vi "Debug Server Launcher.vi"() -> ()   [LabVIEW 2017]
doc: "Splash screen for the Debug Server application"
panel:
  out "dot3 4":picture
  out "dot2 4":picture
  out "dot1 4":picture
  out "dot3 3":picture
  out "dot2 3":picture
  out "dot1 3":picture
  out "dot3 2":picture
  out "dot2 2":picture
  out "dot1 2":picture
  out "dot1":picture
  out "dot2":picture
  out "dot3":picture
  in  "error in (no error)":errorcluster
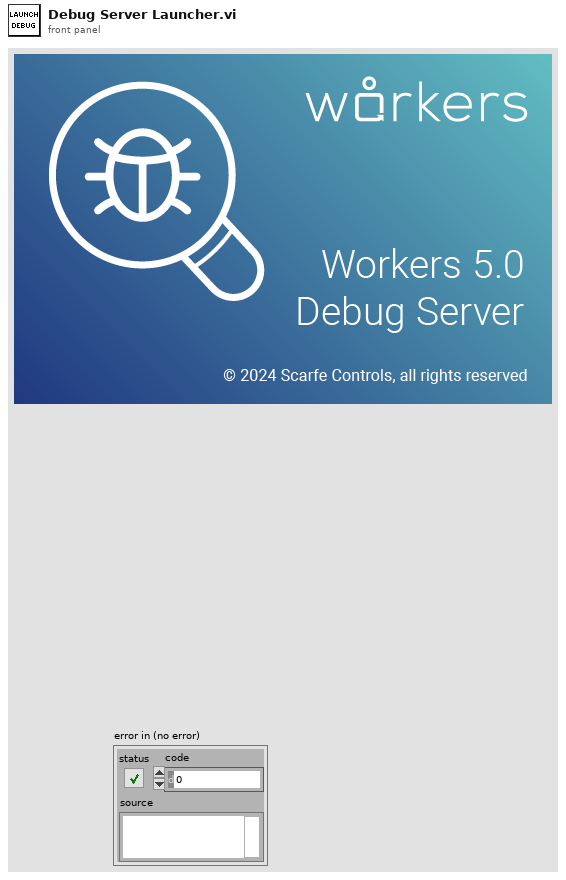
[diagram p1: front panel]
types:
  T1 = enum32{"Invalid", "Standard", "Closed", "Hidden", "Minimized", "Maximized"}
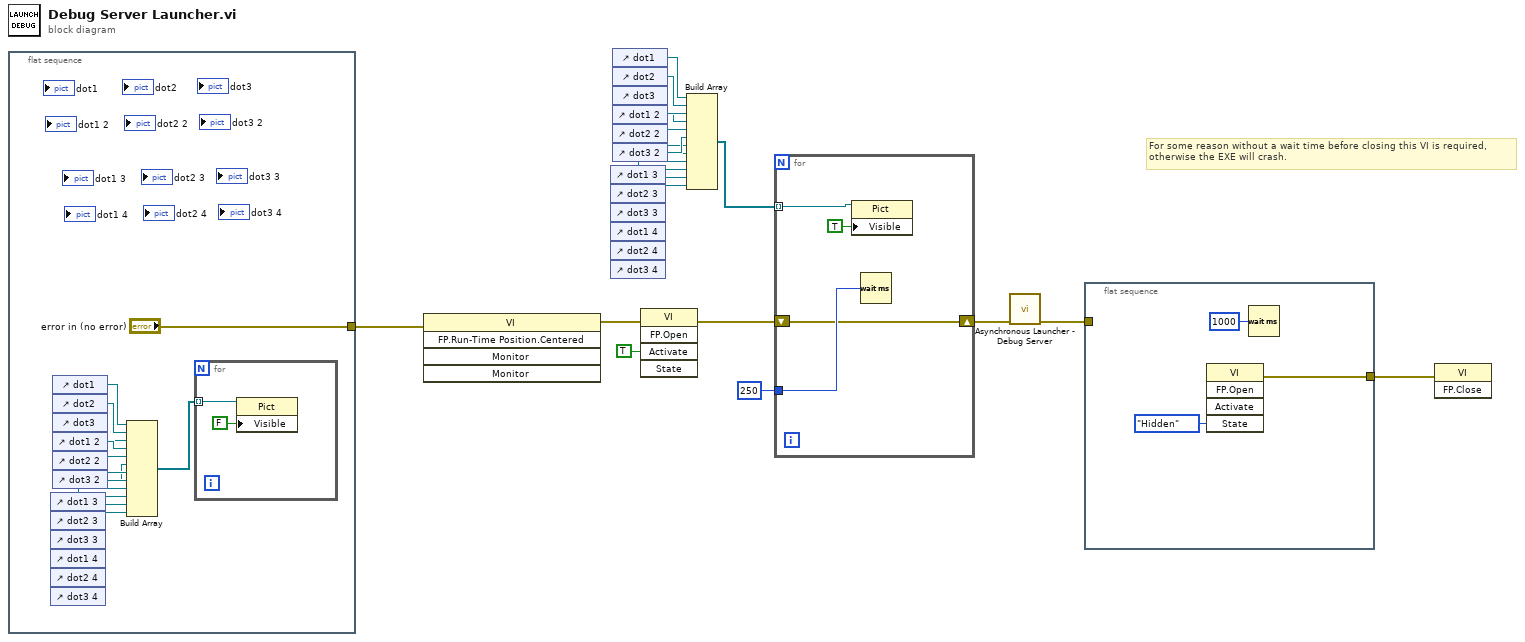
[diagram p0: block diagram]
diagram:
  # "For some reason without a wait time before closing this VI is required,\notherwise the EXE will crash."
  n1 = flat-sequence {
    tunnel: ["error in (no error)"] -> w21
    frame #0 {
      n2 = control-ref of="dot1 3"() -> (w29:refnum<vi>)
      n3 = control-ref of="dot2 3"() -> (w30:refnum<vi>)
      n4 = control-ref of="dot3 3"() -> (w31:refnum<vi>)
      n5 = control-ref of="dot1 4"() -> (w32:refnum<vi>)
      n6 = control-ref of="dot2 4"() -> (w33:refnum<vi>)
      n7 = control-ref of="dot3 4"() -> (w34:refnum<vi>)
      n8 = control-ref of="dot1"() -> (w23:refnum<vi>)
      n9 = control-ref of="dot2"() -> (w24:refnum<vi>)
      n10 = control-ref of="dot3"() -> (w25:refnum<vi>)
      n11 = control-ref of="dot1 2"() -> (w26:refnum<vi>)
      n12 = control-ref of="dot2 2"() -> (w27:refnum<vi>)
      n13 = control-ref of="dot3 2"() -> (w28:refnum<vi>)
      n14 = Build Array(w23, w24, w25, w26, w27, w28, w29, w30, w31, w32, w33, w34) -> (w22:refnum<vi>[])
      n15 = for {
        tunnel: w22 -> [w36] mode=indexing
        n16 = property class="Pict"(reference=w36, "Visible"=FALSE) -> ()  [unwired: 1 in, 2 out]
      }
    }
  }
  n17 = invoke class="VI" method="FP.Run-Time Position.Centered"(error in=w21) -> (error out=w20:errorcluster)  [unwired: 4 in, 4 out]
  n18 = control-ref of="dot1 3"() -> (w8:refnum<vi>)
  n19 = control-ref of="dot2 3"() -> (w7:refnum<vi>)
  n20 = control-ref of="dot3 3"() -> (w6:refnum<vi>)
  n21 = control-ref of="dot1 4"() -> (w5:refnum<vi>)
  n22 = control-ref of="dot2 4"() -> (w4:refnum<vi>)
  n23 = control-ref of="dot3 4"() -> (w3:refnum<vi>)
  n24 = control-ref of="dot1"() -> (w16:refnum<vi>)
  n25 = control-ref of="dot2"() -> (w15:refnum<vi>)
  n26 = control-ref of="dot3"() -> (w14:refnum<vi>)
  n27 = control-ref of="dot1 2"() -> (w13:refnum<vi>)
  n28 = control-ref of="dot2 2"() -> (w12:refnum<vi>)
  n29 = control-ref of="dot3 2"() -> (w11:refnum<vi>)
  n30 = invoke class="VI" method="FP.Open"(error in=w20, "Activate"=TRUE ("Activate?")) -> (error out=w9:errorcluster)  [unwired: 3 in, 4 out]
  n31 = Build Array(w16, w15, w14, w13, w12, w11, w8, w7, w6, w5, w4, w3) -> (w10:refnum<vi>[])
  n32 = for {
    tunnel: u32 250 ("milliseconds to wait") -> [w41]
    tunnel: w10 -> [w39] mode=indexing
    shift-right: [w38] -> w2
    shift-left: w9 -> [w38]
    n33 = property class="Pict"(reference=w39, "Visible"=TRUE) -> ()  [unwired: 1 in, 2 out]
    n34 = Wait (ms)(milliseconds to wait=w41) -> ()  [unwired: 1 out]
  }
  n35 = call "Asynchronous Launcher - Debug Server.vi"("error in"=w2) -> ("error out"=w1:errorcluster)  [unwired: 9 in, 1 out]
  n36 = flat-sequence {
    tunnel: [w43] -> w17
    tunnel: w1 -> [_]
    frame #0 {
      n37 = invoke class="VI" method="FP.Open"("State"=T1."Hidden") -> (error out=w43:errorcluster)  [unwired: 4 in, 4 out]
      n38 = Wait (ms)(milliseconds to wait=u32 1000) -> ()  [unwired: 1 out]
    }
  }
  n39 = invoke class="VI" method="FP.Close"(error in=w17) -> ()  [unwired: 2 in, 3 out]
